vi "local-main.vi"() -> ()   [LabVIEW 2018]
uses:
  <vilib>/MakerHub/Xbox-One-Controller/Public/Open First Controller.vi
  <vilib>/MakerHub/Xbox-One-Controller/LMH-Xbox-One-Controller.lvlib
panel:
  in  "stop":bool
  in  "Reverse y-axis?":bool=TRUE
  in  "Reverse x-axis?":bool=TRUE
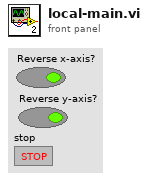
[diagram p1: front panel]
types:
  T1 = typedef "LMH-Xbox-One-Controller.lvlib/Xbox One Controller Ref.ctl" = cluster{"Controller Ref":refnum<k1>, "Event Refnum":refnum<event-registration>, "Worker Ref":refnum<vi>}
  T2 = typedef "LMH-Xbox-One-Controller.lvlib/All Axis Data.ctl" = cluster{"Left Stick":cluster{"X Axis":i32, "Y Axis":i32}, "Right Stick":cluster{"X Axis":i32, "Y Axis":i32}, "Triggers":i32, "D-Pad":T3}
  T3 = typedef "LMH-Xbox-One-Controller.lvlib/DPad Enum.ctl" = enum16{"Idle", "Up", "Up / Right", "Right", "Down / Right", "Down", "Down / Left", "Left", "Up / Left"}
  T4 = typedef "LMH-Xbox-One-Controller.lvlib/All Buttons Visual.ctl" = cluster{"A":T5, "B":T6, "X":T7, "Y":T8, "Left Bumper":T9, "Right Bumper":T10, "View Button":T11, "Menu Button":T12, "Left Stick":T13, "Right Stick":T13}
  T5 = typedef "LMH-Xbox-One-Controller.lvlib/A.ctl" = bool
  T6 = typedef "LMH-Xbox-One-Controller.lvlib/B.ctl" = bool
  T7 = typedef "LMH-Xbox-One-Controller.lvlib/X.ctl" = bool
  T8 = typedef "LMH-Xbox-One-Controller.lvlib/Y.ctl" = bool
  T9 = typedef "LMH-Xbox-One-Controller.lvlib/Left Bumper.ctl" = bool
  T10 = typedef "LMH-Xbox-One-Controller.lvlib/Right Bumper.ctl" = bool
  T11 = typedef "LMH-Xbox-One-Controller.lvlib/View.ctl" = bool
  T12 = typedef "LMH-Xbox-One-Controller.lvlib/Menu.ctl" = bool
  T13 = typedef "LMH-Xbox-One-Controller.lvlib/Thumbstick.ctl" = bool
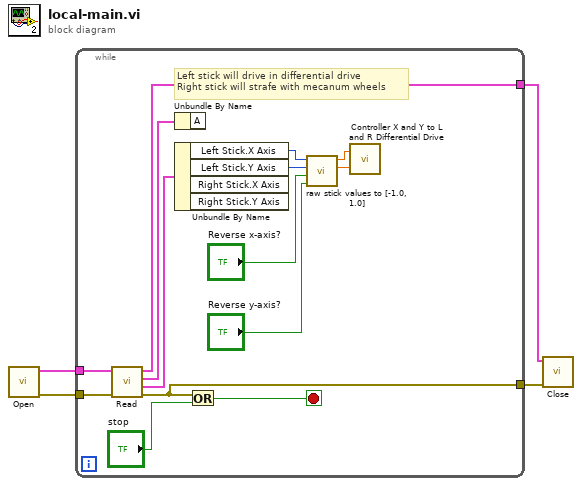
[diagram p0: block diagram]
diagram:
  n1 = call-poly <vilib>:"Open.vi"() -> ("Error Out"=w3:errorcluster, "Xbox One Controller"=w4:T1)  [unwired: 9 in, 1 out]
  n2 = while {
    tunnel: w4 -> [w18]
    tunnel: w3 -> [w17]
    tunnel: [w16] -> w2
    tunnel: [w5] -> w1
    stop <- w6 stop-if-true
    # "Left stick will drive in differential drive\nRight stick will strafe with mecanum wheels"
    n3 = call <vilib>:"Read.vi"("Error In"=w17, "Xbox One Controller Ref"=w18) -> ("Error Out"=w5:errorcluster, "All Axis"=w14:T2, "Buttons"=w15:T4, "Xbox One Controller Ref"=w16:T1)  [unwired: 6 in]
    n4 = Unbundle By Name(w15) -> ()  [unwired: 1 out]
    n5 = Unbundle By Name(w14) -> ("Left Stick.X Axis"=w13:i32, "Left Stick.Y Axis"=w12:i32)  [unwired: 2 out]
    n6 = Or(x=w5, y="stop") -> (x .or. y?=w6:bool)
    n7 = call "raw stick values to [-1.0, 1.0].vi"("Reverse y-axis?"="Reverse y-axis?", "Reverse x-axis?"="Reverse x-axis?", "raw y-axis"=w12, "raw x-axis"=w13) -> ("normalized y-axis"=w8:dbl, "normalized x-axis"=w9:dbl)  [unwired: 5 in]
    n8 = call "Controller X and Y to L and R Differential Drive.vi"("Controller Y-Axis"=w8, "Controller X-Axis"=w9) -> ()  [unwired: 2 out]
  }
  n9 = call <vilib>:"Close.vi"("Error In"=w1, "Xbox One Controller Ref"=w2) -> ()  [unwired: 9 in, 1 out]
